vi "tcp_io.vi"(0 "Offline queue":refnum<queue>, 1 "Modulation info":T1 {"Hi channels at low" min=0 step=1; "Low carriers" format="%#_6p"; "High carriers" format="%#_6p"}, 2 "Config":T2={"IO params"={"Conversion"={"Rate"=0.0, "Num cards"=0, "Out channels"=0}, "Carriers"={"Phase shift"=0.0, "Levels"=[], "Delay samples"=0.0}, "TCP"={"Host"="192.168.1.15", "Port"=6666, "Buffering"=6, "Timeout"=6}, "Input channel sign"=[1, 1, 1]}, "High rate STFT"={"Win param"=0.0, "Window type"=0, "Win order"=0, "DFT size"=0, "Channels"=[], "Oversample"=0}, "Low rate STFT"={"Win param"=0.0, "Window type"=0, "Win order"=0, "DFT size"=0, "Channels"=[], "Oversample"=0}, "Filtering "=[]} {"Filtering"."Distortion"."Limit" format="%#_3p"; "Filtering"."Distortion"."LF cut" format="%#_3p"; "Filtering"."Kalman"."Measure noise" format="%#_3p"; "Filtering"."Kalman"."Process noise" format="%#_3p"; "Filtering"."Hum"."Limit" format="%#_3p"; "Filtering"."Hum"."Frequency" format="%#_4p"; "Low rate STFT"."Oversample" min=1 step=1; "Low rate STFT"."Channels" min=0 step=1; "Low rate STFT"."DFT size" min=1 step=1; "Low rate STFT"."Window type" items=["Rectangle"=0, "Hanning"=1, "Hamming"=2, "Blackman-Harris"=3, "Exact Blackman"=4, "Blackman"=5, "Flat Top"=6, "4 Term B-Harris "=7, "7 Term B-Harris"=8, "Low Sidelobe"=9, "Blackman Nuttall"=11, "Triangle"=30, "Bartlett-Hanning"=31, "Bohman"=32, "Parzen"=33, "Welch"=34, "Kaiser"=60, "Dolph-Chebyshev"=61, "Gaussian"=62]; "High rate STFT"."Oversample" min=1 step=1; "High rate STFT"."Channels" min=0 step=1; "High rate STFT"."DFT size" min=1 step=1; "High rate STFT"."Window type" items=["Rectangle"=0, "Hanning"=1, "Hamming"=2, "Blackman-Harris"=3, "Exact Blackman"=4, "Blackman"=5, "Flat Top"=6, "4 Term B-Harris "=7, "7 Term B-Harris"=8, "Low Sidelobe"=9, "Blackman Nuttall"=11, "Triangle"=30, "Bartlett-Hanning"=31, "Bohman"=32, "Parzen"=33, "Welch"=34, "Kaiser"=60, "Dolph-Chebyshev"=61, "Gaussian"=62]; "IO params"."Input channel sign" min=-1 max=1 step=1; "IO params"."Carriers"."Levels" min=0.0 step=0.1; "IO params"."Conversion"."Rate" format="%#_8g"}, 5 "Read queue":refnum<queue>, 9 "Freq response":bool, 11 "Connection in":refnum<k5>, 12 "Write sequence":i32, 13 "Offline":bool) -> (3 "Read backlog":i32, 4 "Backlog":bool, 6 "Connection out":refnum<k5>, 8 "Source waveforms":waveform(dbl)[](graph), 10 "Restart IO":bool, 14 "Comp fault":bool, 15 "error out":errorcluster)   [LabVIEW 2026]
uses:
  processing/ilemt_config.ctl
  IO_params.ctl
  processing/stft_params.ctl
  <vilib>/Analysis/4window.llb/windowTd.ctl
  processing/filter_params.ctl
  processing/detrend_mode.ctl
  processing/modulation_info.ctl
  <vilib>/Analysis/NI_AALPro.lvlib
panel:
  out "Sequence diff":u8
  out "Read sequence":u8
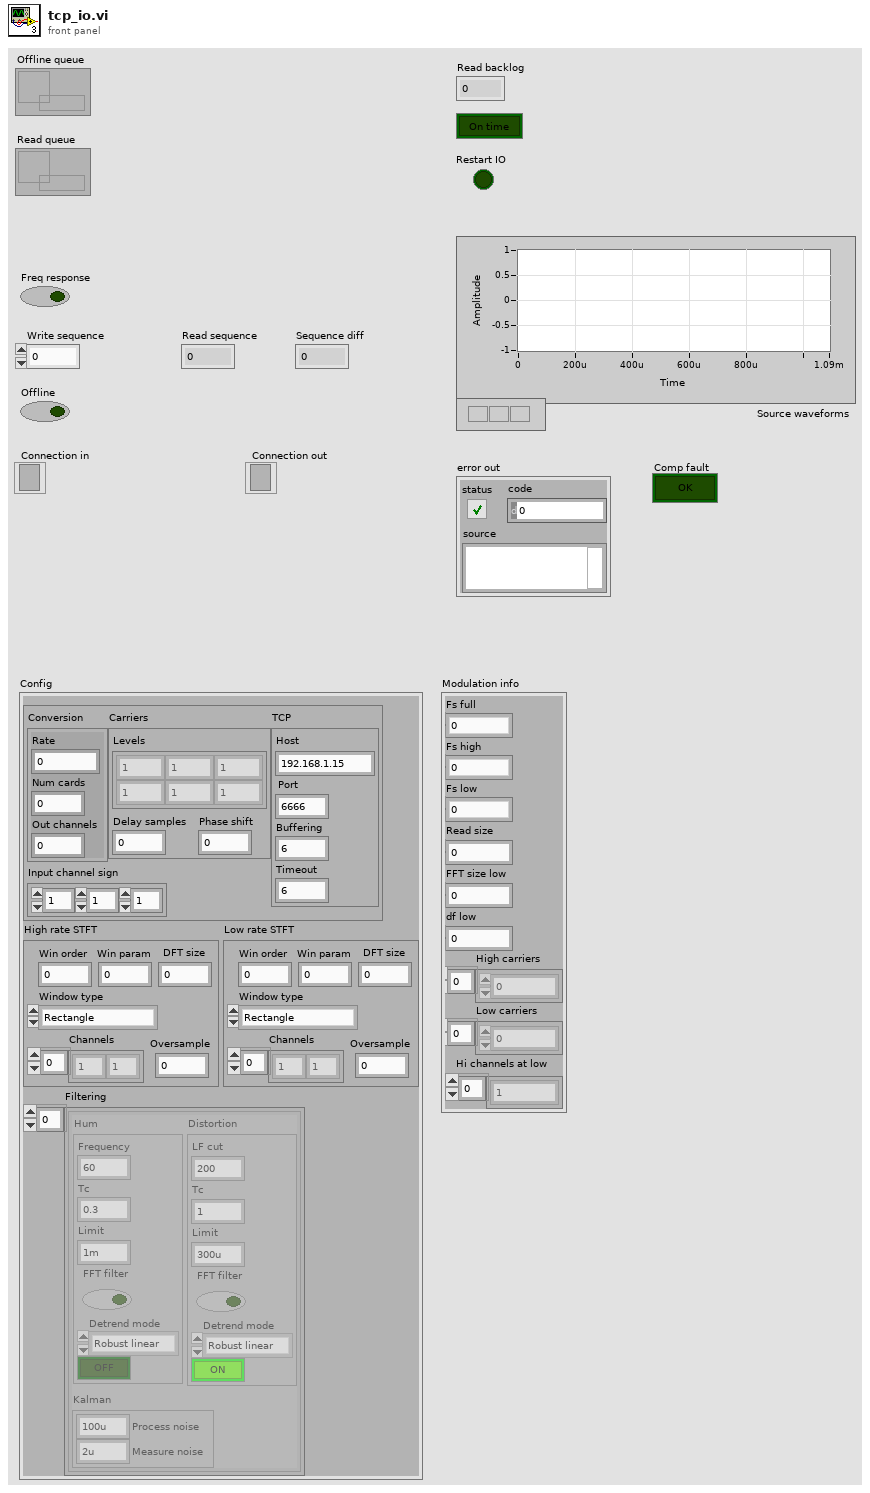
[diagram p1: front panel]
types:
  T1 = typedef "modulation_info.ctl" = cluster{"Fs full":dbl, "Fs high":dbl, "Fs low":dbl, "Read size":i32, "FFT size low":i32, "df low":dbl, "High carriers":dbl[], "Low carriers":dbl[], "Hi channels at low":i32[]}
  T2 = typedef "ilemt_config.ctl" = cluster{"IO params":T3, "High rate STFT":T4, "Low rate STFT":T4, "Filtering ":T6[]}
  T3 = typedef "IO_params.ctl" = cluster{"Conversion":cluster{"Rate":dbl, "Num cards":u32, "Out channels":u32}, "Carriers":cluster{"Phase shift":dbl, "Levels":dbl[][], "Delay samples":dbl}, "TCP":cluster{"Host":string, "Port":i32, "Buffering":u32, "Timeout":u32}, "Input channel sign":i32[]}
  T4 = typedef "stft_params.ctl" = cluster{"Win param":dbl, "Window type":T5, "Win order":i32, "DFT size":i32, "Channels":i32[], "Oversample":i32}
  T5 = typedef "NI_AALPro.lvlib/windowTd.ctl" = u32
  T6 = typedef "filter_params.ctl" = cluster{"Hum":cluster{"Frequency":dbl, "Tc":dbl, "Limit":dbl, "FFT filter":bool, "Detrend mode":T7, "Enable":bool}, "Kalman":cluster{"Process noise":dbl, "Measure noise":dbl}, "Distortion":cluster{"LF cut":dbl, "Tc":dbl, "Limit":dbl, "FFT filter":bool, "Detrend mode":T7, "Enable":bool}}
  T7 = typedef "detrend_mode.ctl" = enum16{"Zero mean", "Linear", "Robust linear"}
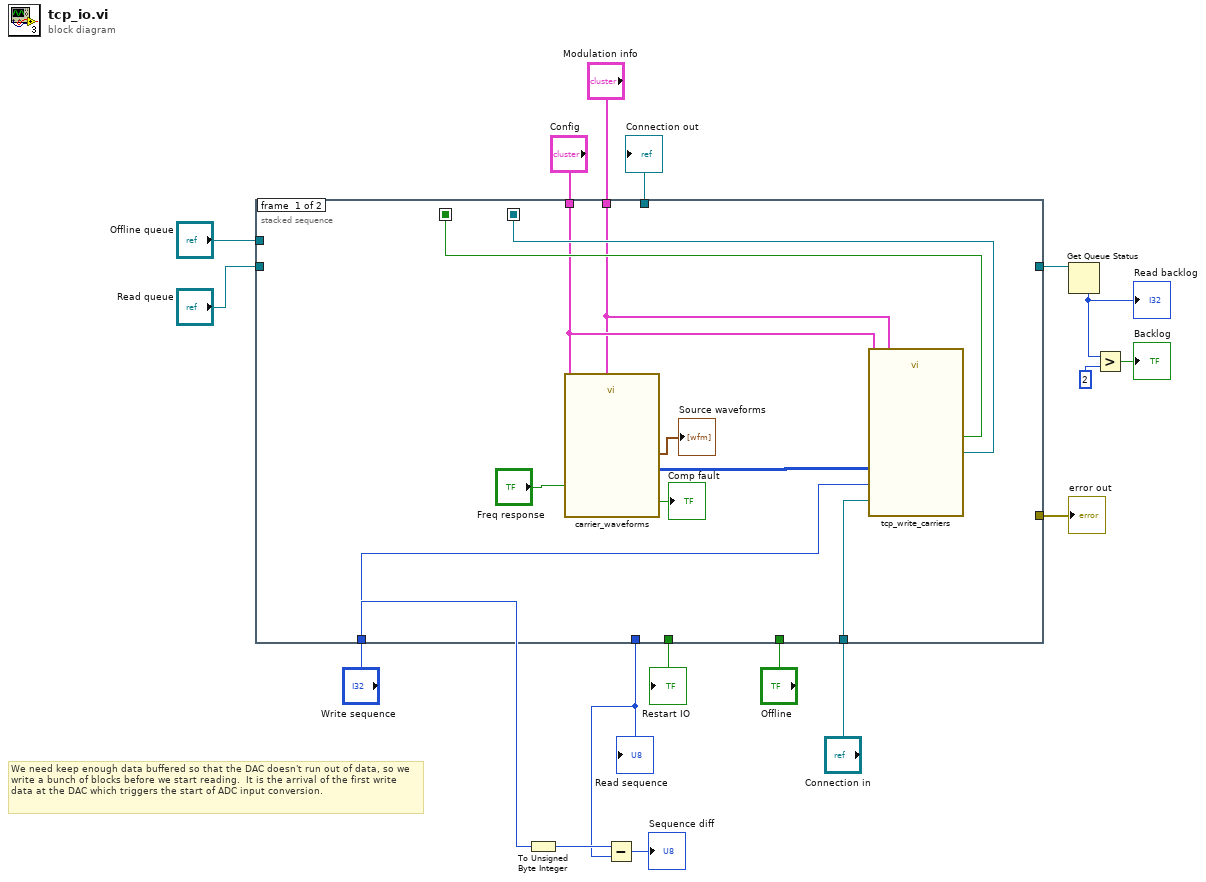
[diagram p0: block diagram]
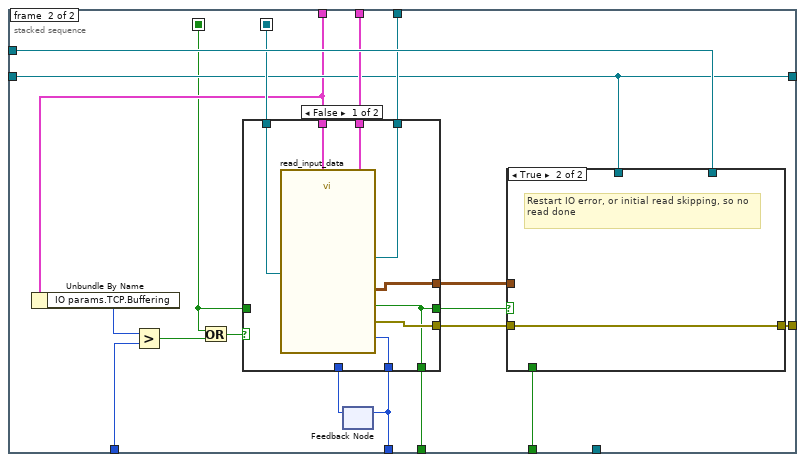
[diagram p2: hidden frame]
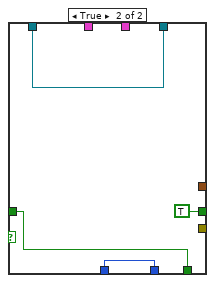
[diagram p3: hidden frame]
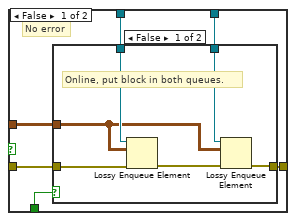
[diagram p4: hidden frame]
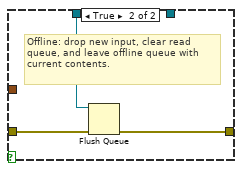
[diagram p5: hidden frame]
diagram:
  # "We need keep enough data buffered so that the DAC doesn't run out of data, so we write a bunch of blocks before we start reading.  It is the arrival of the first write data at the DAC which triggers the start of ADC input conversion."
  n1 = stacked-sequence {
    seq-local: [w24 _] -> [_ w40]
    seq-local: [w21 _] -> [_ w31]
    tunnel: "Read queue" -> [_ w37]
    tunnel: "Offline queue" -> [_ w46]
    tunnel: "Modulation info" -> [w19 w41]
    tunnel: [_ w44] -> w16
    tunnel: "Write sequence" -> [w26 w36]
    tunnel: "Config" -> [w20 w34]
    tunnel: "Offline" -> [_ w43]
    tunnel: "Connection in" -> [w23 _]
    tunnel: [_ w39] -> w12
    tunnel: [_ w38] -> w11
    tunnel: [_ w37] -> w6
    tunnel: [_ w28] -> w1
    frame #0 {
      n2 = call "carrier_waveforms.vi"("Modulation info"=w19, "Freq response"="Freq response", "ilemt_config"=w20) -> ("Comp fault"=→"Comp fault":bool, "Output data"=w22:i32[][], "Source waveforms"=→"Source waveforms":waveform(dbl)[])  [unwired: 6 in]
      n3 = call "tcp_write_carriers.vi"("Modulation info"=w19, "ilemt_config"=w20, "Sequence"=w26, "Carrier output"=w22, "Connection in"=w23) -> ("Restart IO"=w21:bool, "Connection out"=w24:refnum<k5>)  [unwired: 5 in]
    }
    frame #1 {
      n4 = Unbundle By Name(w34) -> ("IO params.TCP.Buffering"=w35:u32)
      n5 = Greater?(x=w35, y=w36) -> (0:w32:bool)
      n6 = Or(x=w31, y=w32) -> (x .or. y?=w33:bool)
      n7 = feedback #1() -> (w29:u8)  [unwired: 1 in]
      n8 = case shown="False" w33 {
        tunnel: [w54 _] -> w45
        tunnel: w34 -> [w53 _]
        tunnel: [w52 _] -> w42
        tunnel: w41 -> [w51 _]
        tunnel: w40 -> [w50 w58]
        tunnel: [w49 w58] -> w39
        tunnel: [w48 w57] -> w38
        tunnel: w31 -> [_ w57]
        tunnel: [w48 TRUE ("Restart IO")] -> w30
        tunnel: [w47 w55] -> w28
        tunnel: w29 -> [_ w55]
        frame False {
          n9 = call "read_input_data.vi"("Modulation info"=w51, "Config"=w53, "Connection in"=w50) -> ("error out"=w54:errorcluster, "Restart IO"=w48:bool, "Input data"=w52:waveform(dbl)[][], "Connection out"=w49:refnum<k5>, "Sequence"=w47:u8)  [unwired: 4 in]
        }
        frame True {
        }
      }
      n10 = feedback-in #1(w28) -> ()
      n11 = case shown="True" w30 {
        tunnel: w37 -> [w64 _]
        tunnel: w46 -> [w63 _]
        tunnel: w45 -> [w62 w74]
        tunnel: [w61 w74] -> w44
        tunnel: w43 -> [w60 _]
        tunnel: w42 -> [w59 _]
        frame False {
          # "No error"
          n12 = case shown="False" w60 {
            tunnel: w62 -> [w70 w72]
            tunnel: w64 -> [w69 w73]
            tunnel: w63 -> [w67 _]
            tunnel: w59 -> [w66 _]
            tunnel: [w65 w71] -> w61
            frame False {
              # "Online, put block in both queues."
              n13 = Lossy Enqueue Element(queue=w69, element=w66, error in (no error)=w70) -> (error out=w68:errorcluster)  [unwired: 3 out]
              n14 = Lossy Enqueue Element(queue=w67, element=w66, error in (no error)=w68) -> (error out=w65:errorcluster)  [unwired: 3 out]
            }
            frame True {
              # "Offline: drop new input, clear read queue, and leave offline queue with current contents."
              n15 = Flush Queue(queue=w73, error in (no error)=w72) -> (error out=w71:errorcluster)  [unwired: 2 out]
            }
          }
        }
        frame True {
          # "Restart IO error, or initial read skipping, so no read done"
        }
      }
    }
  }
  "error out" <- w16
  "Connection out" <- w12
  "Restart IO" <- w11
  "Read sequence" <- w1
  n16 = To Unsigned Byte Integer(number="Write sequence") -> (unsigned 8bit integer=w3:u8)
  n17 = Subtract(x=w3, y=w1) -> (x-y=→"Sequence diff":u8)
  n18 = Get Queue Status(queue=w6) -> (# elements in queue=w9:i32)  [unwired: 2 in, 7 out]
  "Read backlog" <- w9
  n19 = Greater?(x=w9, y=2) -> (0:→"Backlog":bool)
